vi "DecayAnalysis.vi"() -> ()   [LabVIEW 2015]
uses:
  <vilib>/gmath/SpecialFunctions.llb/Factorial.vi
  <vilib>/Utility/file.llb/Read Delimited Spreadsheet (DBL).vi
  <vilib>/imath/engines/lvmath2/RunTimeEngine/Managers/WorkSpace/UID Generator.vi
  <vilib>/imath/engines/lvmath2/RunTimeEngine/BuiltInFunctions/size/NIMS_I32Row=size(GM).vi
  <instcachedir>/0/NIMS_I32Row=size(GM)_10ACDCB9F1F84A7E9F42C91D87611FB5.lvgen/NIMS_I32Row=size(GM)_10ACDCB9F1F84A7E9F42C91D87611FB5_001.vi
  <vilib>/imath/engines/lvmath2/RunTimeEngine/RunTimeType/NIMS_RunTimeType_From StrictType (excl LVString).vi
  <instcachedir>/0/NIMS_RunTimeType_From StrictType (excl LVString)_EB1C38A9BC5048DA9ABDA8F781E54D21.lvgen/NIMS_RunTimeType_From StrictType (excl LVString)_EB1C38A9BC5048DA9ABDA8F781E54D21_000.vi
  <vilib>/imath/engines/lvmath2/RunTimeEngine/LocalVariableDefStatement/MC_LocalVariableDefStatement_Display.vi
  <vilib>/imath/engines/lvmath2/RunTimeEngine/IndexRead/NIMS M(S,S).vi
  <instcachedir>/0/NIMS M(S,S)_AC51E74150A542F7991B9634C66F3096.lvgen/NIMS M(S,S)_AC51E74150A542F7991B9634C66F3096_002.vi
  <vilib>/imathl/engines/lvmath/Functions/Error Handling/Create Error.vi
  <vilib>/imath/engines/lvmath2/RunTimeEngine/IndexRead/NIMS M(S,R2).vi
  <instcachedir>/0/NIMS M(S,R2)_45730E4D0DB74D118F715F4F99DCE4D7.lvgen/NIMS M(S,R2)_45730E4D0DB74D118F715F4F99DCE4D7_000.vi
  <vilib>/imath/engines/lvmath2/RunTimeEngine/Managers/SymbolTable/Clear UID.vi
  <vilib>/imath/engines/lvmath2/RunTimeEngine/NodeEndStatement/NIMS_NodeEndStatement_Output.vi
  <instcachedir>/0/NIMS_NodeEndStatement_Output_53EC0D466D134D7ABD903AC30B43404B.lvgen/NIMS_NodeEndStatement_Output_53EC0D466D134D7ABD903AC30B43404B_004.vi
  <instcachedir>/0/NIMS_NodeEndStatement_Output_53EC0D466D134D7ABD903AC30B43404B.lvgen/NIMS_NodeEndStatement_Output_53EC0D466D134D7ABD903AC30B43404B_005.vi
  <vilib>/imath/engines/lvmath2/RunTimeEngine/ErrorHandling/NIMS_Finalize Error.vi
  <vilib>/imath/engines/lvmath2/RunTimeEngine/BuiltInFunctions/size/NIMS_I32Row=size(GRow).vi
  <instcachedir>/0/NIMS_I32Row=size(GRow)_E5C05C6B13124B29B774CC4F993D3C59.lvgen/NIMS_I32Row=size(GRow)_E5C05C6B13124B29B774CC4F993D3C59_000.vi
  <vilib>/imath/engines/lvmath2/RunTimeEngine/RangeToken/NIMS_Range_R3 - Integer.vi
  <instcachedir>/0/NIMS_Range_R3 - Integer_366A129248D04497B137BFE8B5AEC90C.lvgen/NIMS_Range_R3 - Integer_366A129248D04497B137BFE8B5AEC90C_000.vi
  <vilib>/imath/engines/lvmath2/RunTimeEngine/CommandStatement/MC_CommandStatement_break.vi
  <instcachedir>/0/NIMS M(S,S)_AC51E74150A542F7991B9634C66F3096.lvgen/NIMS M(S,S)_AC51E74150A542F7991B9634C66F3096_000.vi
  <vilib>/imath/engines/lvmath2/RunTimeEngine/ErrorHandling/NIMS_Create Error From Enums.vi
  <vilib>/imath/engines/lvmath2/RunTimeEngine/BuiltInFunctions/power/NIMS_power.vi
  <instcachedir>/0/NIMS_power_DE9EF8C474204F82B150926BE18EE080.lvgen/NIMS_power_DE9EF8C474204F82B150926BE18EE080_000.vi
  <instcachedir>/0/NIMS_power_DE9EF8C474204F82B150926BE18EE080.lvgen/NIMS_power_DE9EF8C474204F82B150926BE18EE080_016.vi
  <vilib>/imath/engines/lvmath2/RunTimeEngine/ArithmeticOperatorToken/NIMS_ArithmeticOperator_rightdiv(C,C).vi
  <instcachedir>/0/NIMS_ArithmeticOperator_rightdiv(C,C)_0424CF3AD6F140AB9AC75AA0AD905D3D.lvgen/NIMS_ArithmeticOperator_rightdiv(C,C)_0424CF3AD6F140AB9AC75AA0AD905D3D_000.vi
  <vilib>/imath/engines/lvmath2/RunTimeEngine/Managers/SymbolTable/NIMS_WorkSpace.lvlib
  <vilib>/Analysis/NI_AALBase.lvlib
  <vilib>/gmath/NI_Gmath.lvlib
panel:
  out "Constant Rate":cluster{"X Values":dbl[], "p":dbl[]}[](graph)
  out "Decay Plot":cluster{"time":i32[], "Array":dbl[]}[](graph)=[{"time"=[50, 51, 52, 53, 54, 55, 56, 57, 58, 59, 60, 61, 62, 63, 64, 65, 66, 67, 68, 69, 70, 71, 72, 73, 74, 75, 76, 77, 78, 79, 80, 81, 82, 83, 84, 85, 86, 87, 88, 89, 90, 91, 92, 93, 94, 95, 96, 97, 98, 99, 100, 101, 102, 103, 104, 105, 106, 107, 108, 109, 110, 111, 112, 113, 114, 115, 116, 117, 118, 119, 120, 121, 122, 123, 124, 125, 126, 127, 128, 129, 130, 131, 132, 133, 134, 135, 136, 137, 138, 139, 140, 141, 142, 143, 144, 145, 146, 147, 148, 149, 150, 151, 152, 153, 154, 155, 156, 157, 158, 159, 160, 161, 162, 163, 164, 165, 166, 167, 168, 169, 170, 171, 172, 173, 174, 175, 176, 177, 178, 179, 180, 181, 182, 183, 184, 185, 186, 187, 188, 189, 190, 191, 192, 193, 194, 195, 196, 197, 198, 199, 200, 201, 202, 203, 204, 205, 206, 207, 208, 209, 210, 211, 212, 213, 214, 215, 216, 217, 218, 219, 220, 221, 222, 223, 224, 225, 226, 227, 228, 229, 230, 231, 232, 233, 234, 235, 236, 237, 238, 239, 240, 241, 242, 243, 244, 245, 246, 247, 248, 249, 250, 251, 252, 253, 254, 255, 256, 257, 258, 259, 260, 261, 262, 263, 264, 265, 266, 267, 268, 269, 270, 271, 272, 273, 274, 275, 276, 277, 278, 279, 280, 281, 282, 283, 284, 285, 286, 287, 288, 289, 290, 291, 292, 293, 294, 295, 296, 297, 298, 299, 300], "Array"=[42.0, 41.0, 55.0, 40.0, 56.0, 52.0, 53.0, 47.0, 50.0, 46.0, 43.0, 54.0, 52.0, 57.0, 42.0, 52.0, 47.0, 57.0, 45.0, 39.0, 48.0, 42.0, 51.0, 51.0, 38.0, 46.0, 45.0, 39.0, 45.0, 42.0, 38.0, 36.0, 47.0, 36.0, 55.0, 38.0, 43.0, 42.0, 34.0, 43.0, 47.0, 39.0, 41.0, 46.0, 52.0, 42.0, 45.0, 33.0, 45.0, 32.0, 37.0, 41.0, 44.0, 33.0, 47.0, 44.0, 51.0, 44.0, 41.0, 53.0, 45.0, 42.0, 32.0, 38.0, 40.0, 29.0, 33.0, 53.0, 38.0, 32.0, 44.0, 46.0, 34.0, 41.0, 41.0, 49.0, 43.0, 37.0, 38.0, 42.0, 37.0, 35.0, 39.0, 41.0, 42.0, 35.0, 45.0, 43.0, 50.0, 36.0, 42.0, 35.0, 39.0, 41.0, 34.0, 36.0, 38.0, 32.0, 37.0, 45.0, 38.0, 36.0, 37.0, 39.0, 27.0, 32.0, 32.0, 38.0, 38.0, 41.0, 41.0, 32.0, 38.0, 39.0, 38.0, 37.0, 39.0, 34.0, 35.0, 41.0, 41.0, 32.0, 39.0, 41.0, 31.0, 40.0, 42.0, 40.0, 41.0, 28.0, 33.0, 39.0, 48.0, 39.0, 43.0, 47.0, 48.0, 40.0, 32.0, 39.0, 37.0, 37.0, 40.0, 42.0, 44.0, 35.0, 40.0, 45.0, 37.0, 38.0, 37.0, 44.0, 35.0, 38.0, 34.0, 43.0, 32.0, 39.0, 38.0, 50.0, 41.0, 44.0, 42.0, 34.0, 34.0, 43.0, 39.0, 35.0, 29.0, 31.0, 37.0, 36.0, 33.0, 37.0, 38.0, 39.0, 24.0, 40.0, 38.0, 33.0, 31.0, 37.0, 36.0, 45.0, 47.0, 40.0, 38.0, 42.0, 35.0, 30.0, 36.0, 41.0, 35.0, 32.0, 32.0, 40.0, 38.0, 48.0, 31.0, 31.0, 35.0, 40.0, 42.0, 44.0, 37.0, 25.0, 41.0, 42.0, 31.0, 36.0, 33.0, 39.0, 26.0, 33.0, 40.0, 29.0, 35.0, 39.0, 44.0, 29.0, 29.0, 35.0, 41.0, 44.0, 37.0, 34.0, 36.0, 31.0, 32.0, 42.0, 33.0, 37.0, 29.0, 32.0, 26.0, 36.0, 26.0, 26.0, 33.0, 48.0, 40.0, 35.0, 31.0, 34.0, 41.0, 36.0, 31.0, 37.0, 35.0, 32.0, 47.0, 34.0]}, {"time"=[50, 51, 52, 53, 54, 55, 56, 57, 58, 59, 60, 61, 62, 63, 64, 65, 66, 67, 68, 69, 70, 71, 72, 73, 74, 75, 76, 77, 78, 79, 80, 81, 82, 83, 84, 85, 86, 87, 88, 89, 90, 91, 92, 93, 94, 95, 96, 97, 98, 99, 100, 101, 102, 103, 104, 105, 106, 107, 108, 109, 110, 111, 112, 113, 114, 115, 116, 117, 118, 119, 120, 121, 122, 123, 124, 125, 126, 127, 128, 129, 130, 131, 132, 133, 134, 135, 136, 137, 138, 139, 140, 141, 142, 143, 144, 145, 146, 147, 148, 149, 150, 151, 152, 153, 154, 155, 156, 157, 158, 159, 160, 161, 162, 163, 164, 165, 166, 167, 168, 169, 170, 171, 172, 173, 174, 175, 176, 177, 178, 179, 180, 181, 182, 183, 184, 185, 186, 187, 188, 189, 190, 191, 192, 193, 194, 195, 196, 197, 198, 199, 200, 201, 202, 203, 204, 205, 206, 207, 208, 209, 210, 211, 212, 213, 214, 215, 216, 217, 218, 219, 220, 221, 222, 223, 224, 225, 226, 227, 228, 229, 230, 231, 232, 233, 234, 235, 236, 237, 238, 239, 240, 241, 242, 243, 244, 245, 246, 247, 248, 249, 250, 251, 252, 253, 254, 255, 256, 257, 258, 259, 260, 261, 262, 263, 264, 265, 266, 267, 268, 269, 270, 271, 272, 273, 274, 275, 276, 277, 278, 279, 280, 281, 282, 283, 284, 285, 286, 287, 288, 289, 290, 291, 292, 293, 294, 295, 296, 297, 298, 299, 300], "Array"=[49.19035632714176, 48.989719157049194, 48.792056084427074, 48.59732302344743, 48.40547654177811, 48.21647385089582, 48.030272796542796, 47.8468318493249, 47.66611009544912, 47.488067227598336, 47.31266353594138, 47.139859899276345, 46.96961777630516, 46.80189919703755, 46.63666675432239, 46.47388359550456, 46.31351341420554, 46.15552044222578, 45.99986944156717, 45.84652569657369, 45.695455006188595, 45.5466236763264, 45.399998512357904, 45.255546811706594, 45.113236356554864, 44.97303540665826, 44.834912692266315, 44.69883740714829, 44.564779201722295, 44.432708176286255, 44.30259487434923, 44.17441027606161, 44.0481257917426, 43.92371325550378, 43.80114491896708, 43.68039344507593, 43.561431901998134, 43.4442337571191, 43.32877287112418, 43.21502349216862, 43.10296025013405, 42.99255815097003, 42.883792571119464, 42.77663925202674, 42.671074294727184, 42.56707415451673, 42.46461563570068, 42.36367588642018, 42.264232393555496, 42.166262977704775, 42.06974578823727, 41.97465929841987, 41.880982300615884, 41.78869390155499, 41.69777351767329, 41.608200870522474, 41.51995598224699, 41.43301917112829, 41.347371047195104, 41.2629925078988, 41.17986473385285, 41.09796918463543, 41.017287594654256, 40.937801969072716, 40.85949457979638, 40.78234796151905, 40.706344907827315, 40.63146846736295, 40.55770194004219, 40.48502887333099, 40.413433058575514, 40.34289852738709, 40.27340954808065, 40.204950622166024, 40.13750648089125, 40.07106208183706, 40.00560260556195, 39.94111345229685, 39.877580238688935, 39.81498879459359, 39.753325159913956, 39.69257558148739, 39.63272651001795, 39.57376459705451, 39.51567669201351, 39.45844983924595, 39.40207127514783, 39.346528425313394, 39.291808901730604, 39.237900500018185, 39.18479119670361, 39.13246914654143, 39.08092267987141, 39.030140300015724, 38.98011068071484, 38.930822663601326, 38.88226525571118, 38.83442762703199, 38.78729910808747, 38.74086918755774, 38.69512750993504, 38.65006387321397, 38.60566822661617, 38.56193066834858, 38.51884144339503, 38.47639094134053, 38.43456969422778, 38.3933683744455, 38.35277779264804, 38.31278889570585, 38.27339276468628, 38.23458061286436, 38.19634378376307, 38.1586737492226, 38.121562107498306, 38.08500058138682, 38.04898101637991, 38.01349537884579, 37.97853575423728, 37.944094345326626, 37.91016347046643, 37.876735561876366, 37.84380316395531, 37.81135893161846, 37.77939562865915, 37.74790612613489, 37.716883400777405, 37.68632053342613, 37.65621070748506, 37.62654720740238, 37.597323417172674, 37.56853281886128, 37.54016899115062, 37.51222560790799, 37.48469643677462, 37.457575337775594, 37.4308562619505, 37.404533250004235, 37.37860043097789, 37.35305202093934, 37.327882321693174, 37.303085719509866, 37.27865668387364, 37.25458976624904, 37.23087959886566, 37.20752089352098, 37.184508440400876, 37.16183710691768, 37.13950183656543, 37.11749764779206, 37.095819632888364, 37.074462956893406, 37.053422856516136, 37.03269463907302, 37.01227368144142, 36.992155429028436, 36.97233539475511, 36.95280915805563, 36.93357236389139, 36.91462072177967, 36.8959500048367, 36.87755604883491, 36.85943475127418, 36.84158207046683, 36.82399402463616, 36.80666669102841, 36.789596205037824, 36.7727787593447, 36.756210603066265, 36.739888040920036, 36.72380743239968, 36.707965190963066, 36.692357783232296, 36.67698172820566, 36.66183359648127, 36.64691000949215, 36.63220763875271, 36.61772320511638, 36.60345347804423, 36.589395274884474, 36.5755454601626, 36.561900944882055, 36.5484586858353, 36.53521568492506, 36.52216898849564, 36.509315686674164, 36.49665291272156, 36.48417784239317, 36.4718876933089, 36.459779724332556, 36.44785123496056, 36.43609956471959, 36.42452209257322, 36.41311623633735, 36.40187945210426, 36.390809233675235, 36.37990311200163, 36.36915865463413, 36.35857346518026, 36.348145182769905, 36.337871481528744, 36.32775007005952, 36.31777869093093, 36.307955120174185, 36.29827716678697, 36.288742672244766, 36.27934951001943, 36.27009558510492, 36.26097883354999, 36.25199722199792, 36.24314874723294, 36.23443143573348, 36.22584334323202, 36.21738255428141, 36.209047181827664, 36.20083536678913, 36.19274527764177, 36.18477511001074, 36.176923086267905, 36.16918745513537, 36.161566491294906, 36.15405849500313, 36.14666179171239, 36.13937473169731, 36.132195689686796, 36.125123064501615, 36.11815527869721, 36.111290778211895, 36.10452803202027, 36.0978655317917, 36.09130179155395, 36.08483534736174, 36.07846475697023, 36.07218859951335, 36.06600547518691, 36.05991400493639, 36.05391283014934, 36.04800061235239, 36.042176032912714, 36.03643779274392, 36.03078461201632, 36.02521522987148, 36.019728404140984, 36.014322911069435, 36.00899754504146, 36.00375111831284, 35.998582460745624, 35.993490419547086, 35.988473859012686, 35.9835316602727, 35.97866272104273, 35.97386595537781]}]
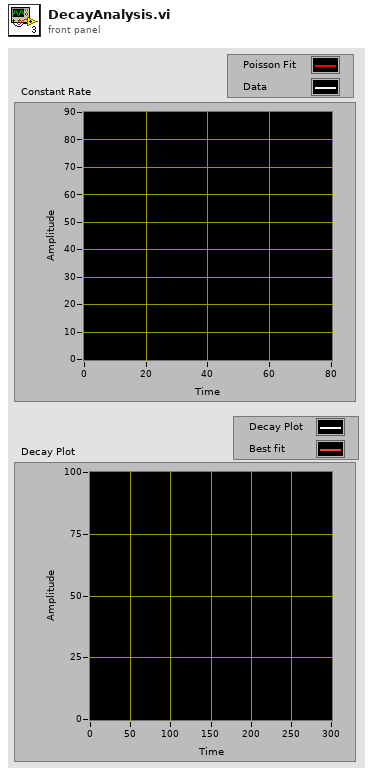
[diagram p1: front panel]
types:
  T1 = cluster{"X Values":dbl[], "Histogram: h(x)":i32[]}
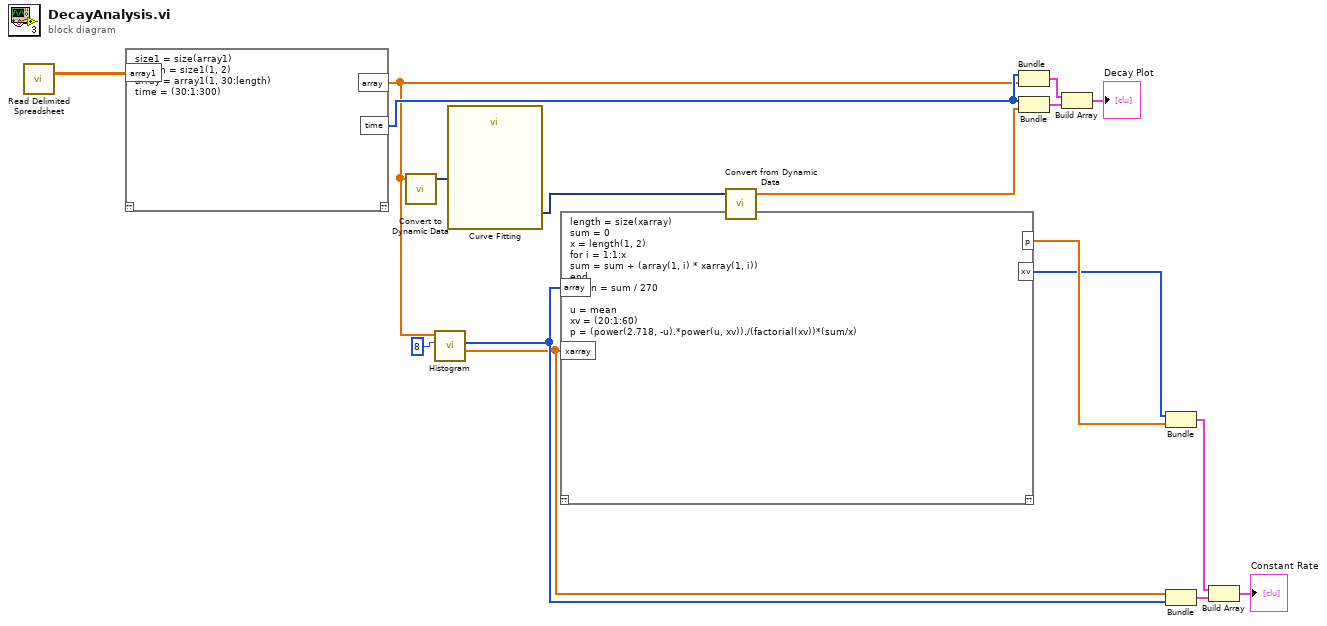
[diagram p0: block diagram]
diagram:
  n1 = call-poly <vilib>:"Read Delimited Spreadsheet.vi"() -> ("all rows"=w1:dbl[][])  [unwired: 10 in, 5 out]
  n2 = mathscript code="size1 = size(array1)\nlength = size1(1, 2)\narray = array1(1, 30:length)\ntime = (30:1:300)"("array1"=w1) -> ("array"=w10:dbl[], "time"=w11:i32[])  [unwired: 1 in, 1 out]
  n3 = call "Convert to Dynamic Data"("Array"=w10) -> ("Dynamic Data Type"=w17:dynamicdata)  [unwired: 3 in]
  n4 = call <vilib>:"Histogram.vi"("intervals"=8, "X"=w10) -> ("X Values"=w7:dbl[], "Histogram: h(x)"=w8:i32[])  [unwired: 6 in, 2 out]
  n5 = call "Curve Fitting"("Signals"=w17) -> ("best fit"=w16:dynamicdata)  [unwired: 6 in, 4 out]
  n6 = mathscript code="length = size(xarray)\nsum = 0\nx = length(1, 2)\nfor i = 1:1:x\nsum = sum + (array(1, i) * xarray(1, i))\nend\nmean = sum / 270\n\nu = mean  \nxv = (20:1:60)\np = (power(2.718, -u).*power(u, xv))./(factorial(xv))*(sum/x)"("array"=w8, "xarray"=w7) -> ("p"=w6:dbl[], "xv"=w2:i32[])  [unwired: 1 in, 1 out]
  n7 = call "Convert from Dynamic Data"("Dynamic Data Type"=w16) -> ("Array"=w15:dbl[])  [unwired: 3 in]
  n8 = Bundle("time"=w11, "array"=w10) -> (w14:cluster{"time":i32[], "array":dbl[]})  [unwired: 1 in]
  n9 = Bundle("time"=w11, "Array"=w15) -> (w13:cluster{"time":i32[], "Array":dbl[]})  [unwired: 1 in]
  n10 = Build Array(w14, w13) -> (→"Decay Plot":cluster{"time":i32[], "Array":dbl[]}[])
  n11 = Bundle("xv"=w2, "p"=w6) -> (w5:cluster{"xv":i32[], "p":dbl[]})  [unwired: 1 in]
  n12 = Bundle("X Values"=w7, "Histogram: h(x)"=w8) -> (w4:T1)  [unwired: 1 in]
  n13 = Build Array(w5, w4) -> (→"Constant Rate":cluster{"X Values":dbl[], "p":dbl[]}[])
